vi "SetParam.vi"(8 "error in (no error)":errorcluster caption="entrée d'erreur (pas d'erreur)", 10 "ParameterSampler":T1={"param_distributions"={"Key"=[], "Value"=[]}, "n_iter"=5, "random_state"=-1} {"random_state" min=-1}, 11 "ParameterSampler.lvclass":refnum<class "ParameterSampler.lvclass">) -> (0 "error out":errorcluster caption="sortie d'erreur", 3 "ParameterSampler.lvclass":refnum<class "ParameterSampler.lvclass">)   [LabVIEW 2020, in "ParameterSampler.lvclass"]
doc: "Set Parameters"
uses:
  ParameterSampler.lvclass
  ParameterSampler.lvclass/ParameterSampler.ctl
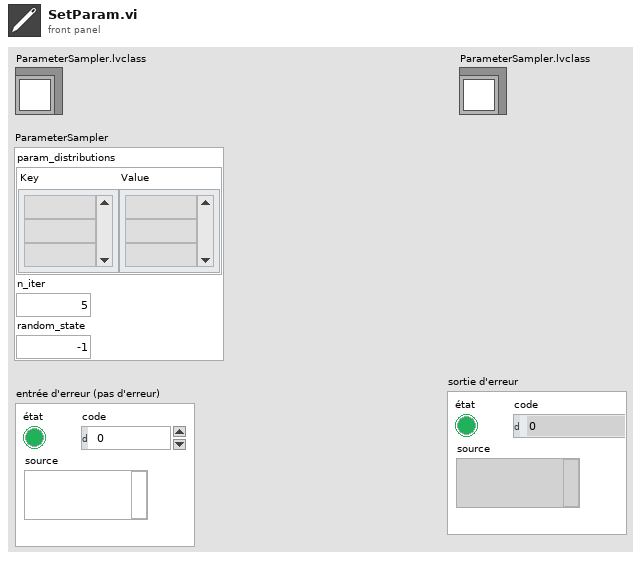
[diagram p1: front panel]
types:
  T1 = cluster{"param_distributions":cluster{"Key":string[], "Value":string[]}, "n_iter":i32, "random_state":i32}
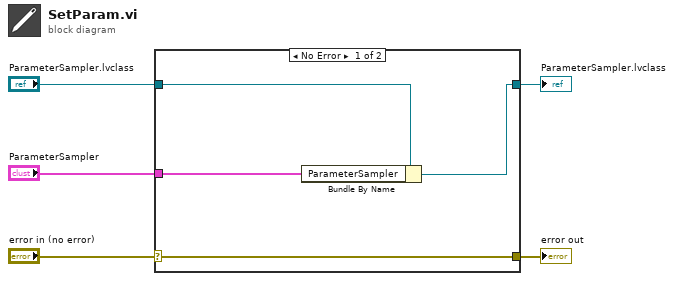
[diagram p0: block diagram]
diagram:
  n1 = case shown="No Error" "error in (no error)" {
    selector: "error in (no error)" -> [w9 w10]
    tunnel: [w9 w10] -> w4
    tunnel: [w7 w11] -> w2
    tunnel: "ParameterSampler.lvclass" -> [w8 w11]
    tunnel: "ParameterSampler" -> [w6 _]
    frame No Error {
      n2 = Bundle By Name(cluster=w8, "ParameterSampler"=w6) -> (w7:refnum<class "ParameterSampler.lvclass">)
    }
    frame Error {
    }
  }
  "error out" <- w4
  "ParameterSampler.lvclass" <- w2
